vi "Integration Query.vi"(8 "error in (no error)":errorcluster, 9 "Wiring (0: 1P2W, 1P2W, 1P2W)":u16(ring) items=["1P2W, 1P2W, 1P2W", "1P3W, 1P2W", "3P3W, 1P2W", "1P2W, 1P3W", "1P2W, 3P3W", "3P4W", "3V3A"], 10 "Element":u8=1 min=1 max=6 step=1, 11 "Yokogawa WT500 in":refnum<class "Yokogawa WT500.lvclass">) -> (0 "error out":errorcluster, 1 "Integration State":T1, 3 "Yokogawa WT500 out":refnum<class "Yokogawa WT500.lvclass">)   [LabVIEW 2014, in "Generic Power Analyzer.lvlib" / "Yokogawa WT500.lvlib" / "Yokogawa WT500.lvclass"]
uses:
  Yokogawa WT500.lvclass
  Universal Power Meter/Universal Power Meter class/Integration State.ctl
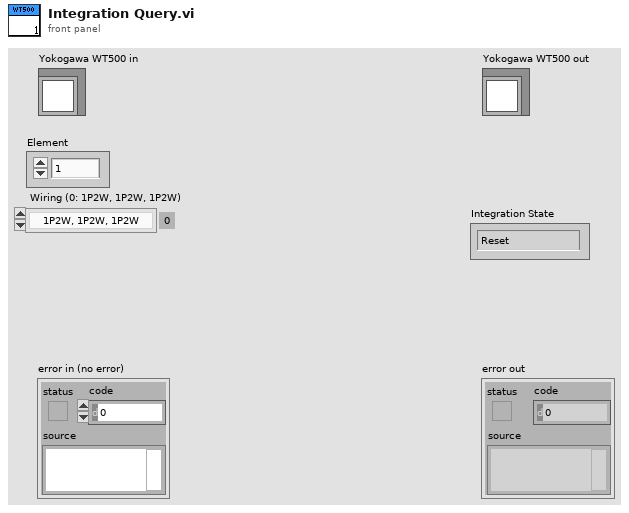
[diagram p1: front panel]
types:
  T1 = typedef "Integration State.ctl" = enum16{"Reset", "Stop", "Start"}
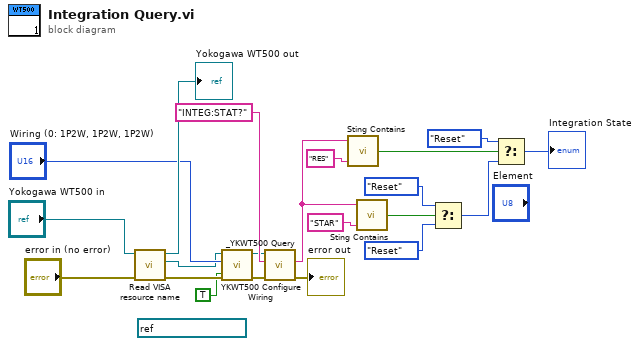
[diagram p0: block diagram]
diagram:
  (unwired) refnum<visa-resource-name> "GPIB0::5::INSTR" ("VISA resource name")
  n1 = call-dynamic "Read VISA resource name.vi"("error in (no error)"="error in (no error)", "Generic Instrument in"="Yokogawa WT500 in") -> ("error out"=w5:errorcluster, "VISA resource name"=w1:refnum<visa-resource-name>, "Generic Instrument out"=→"Yokogawa WT500 out":refnum<class "Yokogawa WT500.lvclass">)  [unwired: 7 in]
  n2 = call <instrlib>:"YKWT500 Configure Wiring.vi"("Enable Independent (False)"=TRUE, "error in (no error)"=w5, "Wiring (0: 1P2W, 1P2W, 1P2W)"="Wiring (0: 1P2W, 1P2W, 1P2W)", "VISA resource name"=w1) -> ("error out"=w6:errorcluster, "VISA resource name out"=w4:refnum<visa-resource-name>)  [unwired: 6 in]
  n3 = call <instrlib>:"_YKWT500 Query.vi"("error in (no error)"=w6, "Write Data"="INTEG:STAT?", "VISA resource name"=w4) -> ("error out"=→"error out":errorcluster, "Read Data"=w7:string)  [unwired: 5 in, 2 out]
  n4 = call "Sting Contains.vi"("Regular expression"="RES" ("Expression to evaluate"), "Input String"=w7) -> ("Boolean"=w17:bool)  [unwired: 3 in]
  n5 = call "Sting Contains.vi"("Regular expression"="STAR" ("Expression to evaluate"), "Input String"=w7) -> ("Boolean"=w15:bool)  [unwired: 3 in]
  n6 = Select(t=Integration_State."Reset" ("Integration State"), s=w15, f=Integration_State."Reset" ("Integration State")) -> (s? t:f=w14:T1)
  n7 = Select(t=Integration_State."Reset" ("Integration State"), s=w17, f=w14) -> (s? t:f=→"Integration State":T1)
